vi "Scott Binary Out.vi"(1 "V- (Not Working":dbl, 2 "V+ (Not Working)":dbl, 3 "Input":i8 min=0 step=1 format="%#.3f") -> ()   [LabVIEW 2012]
uses:
  <vilib>/DAQmx/write.llb/DAQmx Write (Digital Bool 1Line 1Point).vi
  <vilib>/DAQmx/create/channels.llb/DAQmx Create Channel (DO-Digital Output).vi
  <vilib>/DAQmx/miscellaneous.llb/DAQmx Fill In Error Info.vi
panel:
  out "Pin 7":bool
  out "Pin 6":bool
  out "Pin 5":bool
  out "Pin 4":bool
  out "Pin 3":bool
  out "Pin 2":bool
  out "Pin 1":bool
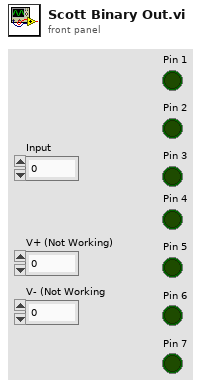
[diagram p1: front panel]
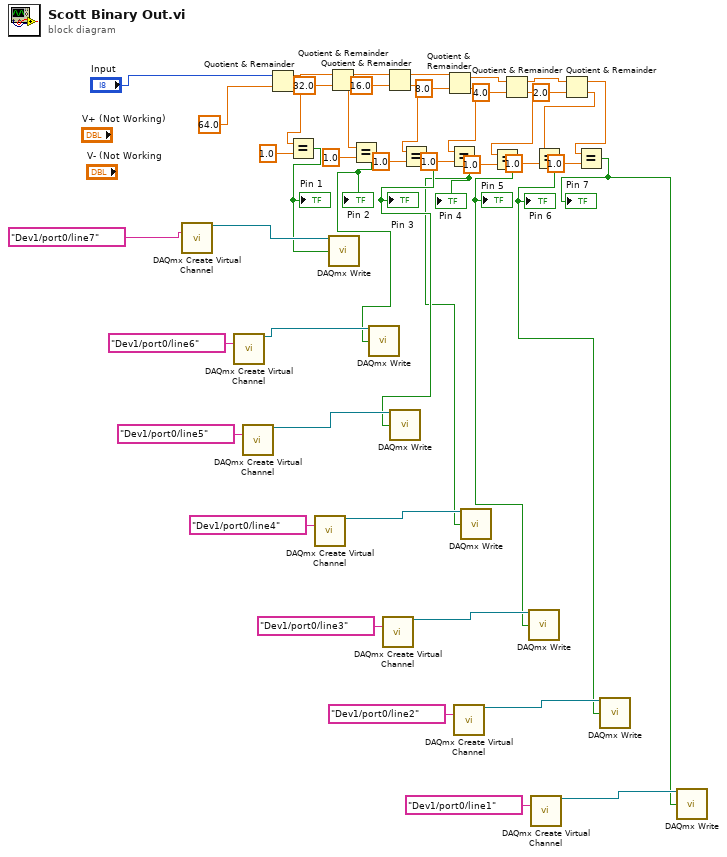
[diagram p0: block diagram]
diagram:
  n1 = call-poly <vilib>:"DAQmx Create Virtual Channel.vi"("lines"=tag "Dev1/port0/line7") -> ("task out"=w21:refnum<k21>)  [unwired: 5 in, 9 out]
  n2 = call-poly <vilib>:"DAQmx Create Virtual Channel.vi"("lines"=tag "Dev1/port0/line6") -> ("task out"=w18:refnum<k21>)  [unwired: 5 in, 9 out]
  n3 = call-poly <vilib>:"DAQmx Create Virtual Channel.vi"("lines"=tag "Dev1/port0/line5") -> ("task out"=w17:refnum<k21>)  [unwired: 5 in, 9 out]
  n4 = Quotient & Remainder(x="Input", y=64.0) -> (x-y*floor(x/y)=w45:dbl, floor(x/y)=w30:dbl)
  n5 = Equal?(x=w30, y=1.0) -> (x = y?=w15:bool)
  "Pin 1" <- w15
  n6 = call-poly <vilib>:"DAQmx Create Virtual Channel.vi"("lines"=tag "Dev1/port0/line4") -> ("task out"=w12:refnum<k21>)  [unwired: 5 in, 9 out]
  n7 = Quotient & Remainder(x=w45, y=32.0) -> (x-y*floor(x/y)=w44:dbl, floor(x/y)=w29:dbl)
  n8 = call-poly <vilib>:"DAQmx Write.vi"("task/channels in"=w21, "data"=w15) -> ()  [unwired: 2 in, 12 out]
  n9 = Equal?(x=w29, y=1.0) -> (x = y?=w14:bool)
  "Pin 2" <- w14
  n10 = call-poly <vilib>:"DAQmx Write.vi"("task/channels in"=w18, "data"=w14) -> ()  [unwired: 2 in, 12 out]
  n11 = call-poly <vilib>:"DAQmx Create Virtual Channel.vi"("lines"=tag "Dev1/port0/line3") -> ("task out"=w10:refnum<k21>)  [unwired: 5 in, 9 out]
  n12 = Quotient & Remainder(x=w44, y=16.0) -> (x-y*floor(x/y)=w43:dbl, floor(x/y)=w28:dbl)
  n13 = Equal?(x=w28, y=1.0) -> (x = y?=w13:bool)
  "Pin 3" <- w13
  n14 = call-poly <vilib>:"DAQmx Write.vi"("task/channels in"=w17, "data"=w13) -> ()  [unwired: 2 in, 12 out]
  n15 = Quotient & Remainder(x=w43, y=8.0) -> (x-y*floor(x/y)=w24:dbl, floor(x/y)=w27:dbl)
  n16 = Equal?(x=w27, y=1.0) -> (x = y?=w4:bool)
  "Pin 4" <- w4
  n17 = call-poly <vilib>:"DAQmx Create Virtual Channel.vi"("lines"=tag "Dev1/port0/line2") -> ("task out"=w8:refnum<k21>)  [unwired: 5 in, 9 out]
  n18 = call-poly <vilib>:"DAQmx Write.vi"("task/channels in"=w12, "data"=w4) -> ()  [unwired: 2 in, 12 out]
  n19 = Quotient & Remainder(x=w24, y=4.0) -> (x-y*floor(x/y)=w23:dbl, floor(x/y)=w26:dbl)
  n20 = Equal?(x=w26, y=1.0) -> (x = y?=w3:bool)
  "Pin 5" <- w3
  n21 = call-poly <vilib>:"DAQmx Write.vi"("task/channels in"=w10, "data"=w3) -> ()  [unwired: 2 in, 12 out]
  n22 = call-poly <vilib>:"DAQmx Create Virtual Channel.vi"("lines"=tag "Dev1/port0/line1") -> ("task out"=w6:refnum<k21>)  [unwired: 5 in, 9 out]
  n23 = Quotient & Remainder(x=w23, y=2.0) -> (x-y*floor(x/y)=w22:dbl, floor(x/y)=w25:dbl)
  n24 = Equal?(x=w25, y=1.0) -> (x = y?=w2:bool)
  "Pin 6" <- w2
  n25 = Equal?(x=w22, y=1.0) -> (x = y?=w1:bool)
  "Pin 7" <- w1
  n26 = call-poly <vilib>:"DAQmx Write.vi"("task/channels in"=w8, "data"=w2) -> ()  [unwired: 2 in, 12 out]
  n27 = call-poly <vilib>:"DAQmx Write.vi"("task/channels in"=w6, "data"=w1) -> ()  [unwired: 2 in, 12 out]
